vi "Init.vi"(8 "error in (no error)":errorcluster, 11 "Data in":refnum<class "DAQmx-Bus.lvclass">) -> (0 "error out":errorcluster, 3 "Data out":refnum<class "DAQmx-Bus.lvclass">)   [LabVIEW 2021, in "DAQmx-Bus.lvclass"]
doc: "Abstract Data Classes 2.1.1.12\nTim Streeter - TSA\nCopyright (c) 2024, TSAOmni-Bus 2.0.1.6\nTim - TSA\nCopyright (c) 2024, TSA"
uses:
  DAQmx-Bus.lvclass
  C:/Program Files (x86)/National Instruments/LabVIEW 2021/vi.lib/TSA/Omni-Bus/Omni-Bus/Bus Access/Bus_Access.lvclass
  <vilib>/TSA/Omni-Bus/Omni-Bus/Bus Access/Bus_Access.lvclass/Bus_Access.ctl
  DAQmx-Bus.lvclass/DAQmx-Bus.ctl
  <vilib>/TSA/Omni-Bus/Omni-Bus/Bus Access/Properties/Read Tag Root.vi
  <vilib>/TSA/Omni-Bus/Omni-Bus/Bus Access/Properties/Write Tags.vi
  <resource>/objmgr/daqmx.rc
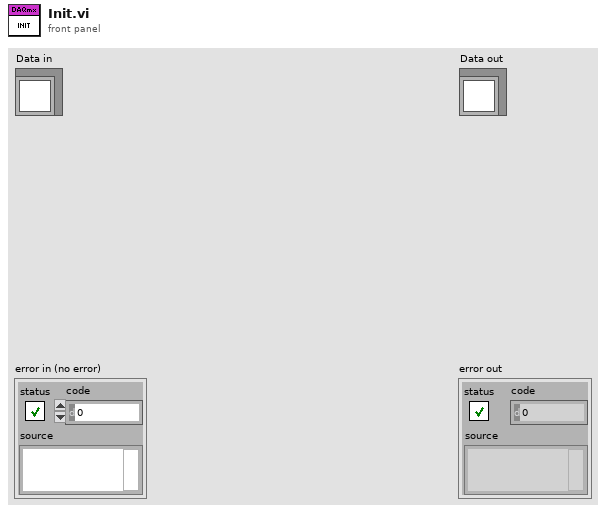
[diagram p1: front panel]
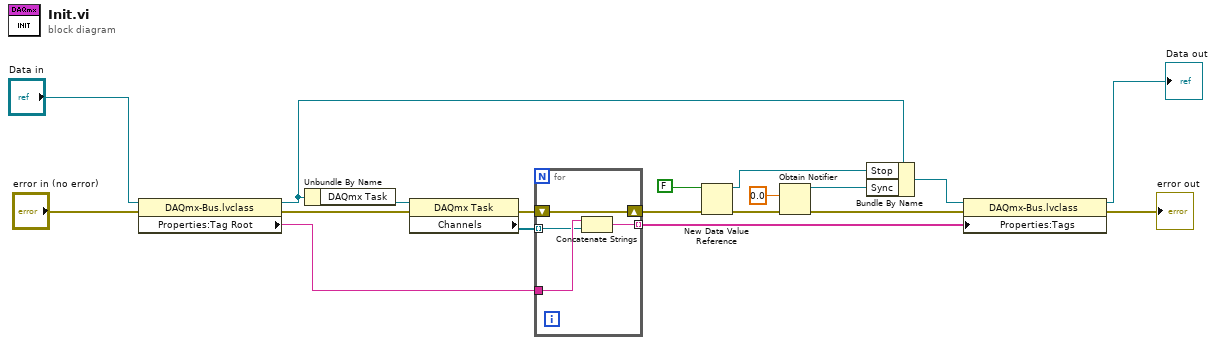
[diagram p0: block diagram]
diagram:
  n1 = property class="DAQmx-Bus.lvclass"(reference="Data in", error in="error in (no error)") -> (reference out=w4:refnum<class "DAQmx-Bus.lvclass">, error out=w7:errorcluster, "Properties:Tag Root"=w3:string)
  n2 = Unbundle By Name(w4) -> ("DAQmx Task"=w19:refnum<k21>)
  n3 = property class="DAQmx Task"(reference=w19, error in=w7) -> (error out=w17:errorcluster, "Channels"=w18:refnum<k21>[])  [unwired: 1 out]
  n4 = for {
    tunnel: w18 -> [w20] mode=indexing
    shift-right: [w23] -> w15
    shift-left: w17 -> [w23]
    tunnel: [w22] -> w2 mode=indexing
    tunnel: w3 -> [w21]
    n5 = Concatenate Strings(w21, w20) -> (w22:string)
  }
  n6 = New Data Value Reference(data value=FALSE, error in=w15) -> (data value reference=w14:refnum<data-value>, error out=w13:errorcluster)
  n7 = Obtain Notifier(notification data type=0.0, error in (no error)=w13) -> (notifier out=w12:refnum<notifier>, error out=w11:errorcluster)  [unwired: 2 in, 1 out]
  n8 = Bundle By Name(cluster=w4, "Stop"=w14, "Sync"=w12) -> (w10:refnum<class "DAQmx-Bus.lvclass">)
  n9 = property class="DAQmx-Bus.lvclass"(reference=w10, error in=w11, "Properties:Tags"=w2) -> (reference out=→"Data out":refnum<class "DAQmx-Bus.lvclass">, error out=→"error out":errorcluster)
